vi "GenerateLeftRight.vi"(10 "TrackWidth":dbl=20.0, 11 "SmoothPath":dbl[][](array[numeric])) -> (1 "Right":dbl[][](array[numeric]), 2 "Left":dbl[][](array[numeric]), 3 "Heading":dbl[](array[numeric]))   [LabVIEW 2016]
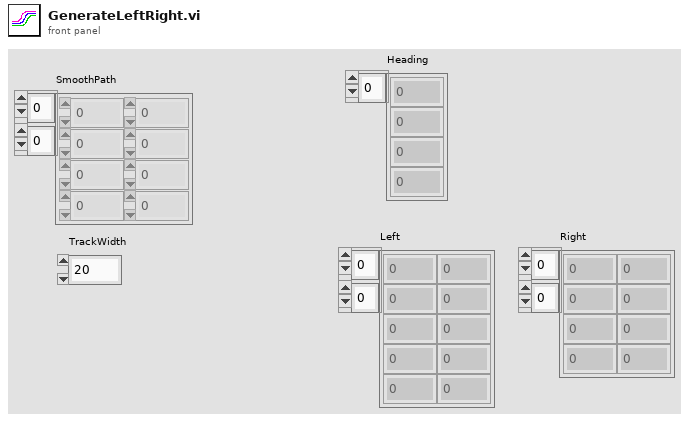
[diagram p1: front panel]
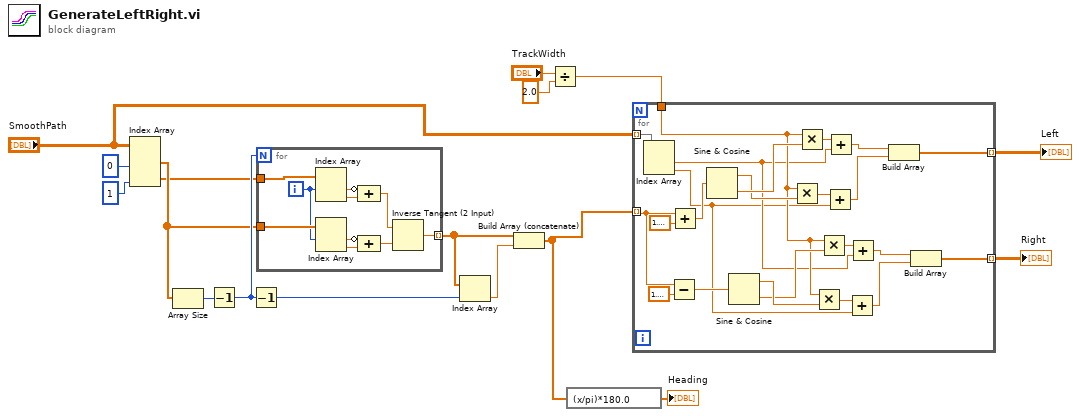
[diagram p0: block diagram]
diagram:
  n1 = Index Array(array="SmoothPath", index (col) #1=0 ("disabled index (col)"), index (col) #2=1 ("index (col)")) -> (element #1=w12:dbl[], element #2=w11:dbl[])  [unwired: 2 in]
  n2 = Array Size(array=w12) -> (size(s)=w16:i32)
  n3 = Decrement(x=w16) -> (x-1=w14:i32)
  n4 = Decrement(x=w14) -> (x-1=w13:i32)
  n5 = for {
    N: w14 -> [_]
    tunnel: w12 -> [w27]
    tunnel: w11 -> [w26]
    tunnel: [w19] -> w3 mode=indexing
    i -> [w18]
    n6 = Index Array(array=w26, index #1=w18) -> (element #1=w24:dbl, element #2=w25:dbl)  [unwired: 1 in]
    n7 = Index Array(array=w27, index #1=w18) -> (element #1=w22:dbl, element #2=w23:dbl)  [unwired: 1 in]
    n8 = Compound Arithmetic op=ADD(invert w24, w25) -> (w21:dbl)
    n9 = Compound Arithmetic op=ADD(invert w22, w23) -> (w20:dbl)
    n10 = Inverse Tangent (2 Input)(1:w20, 2:w21) -> (0:w19:dbl)
  }
  n11 = Index Array(array=w3, index=w13) -> (element=w2:dbl)
  n12 = Build Array (concatenate)(w3, w2) -> (w1:dbl[])
  n13 = Divide(x="TrackWidth", y=2.0) -> (x/y=w8:dbl)
  n14 = expression code="(x/pi)*180.0" ("radians to degrees")(w1) -> (→"Heading":dbl[])
  n15 = for {
    tunnel: w1 -> [w32] mode=indexing
    tunnel: w8 -> [w31]
    tunnel: "SmoothPath" -> [w33] mode=indexing
    tunnel: [w42] -> w6 mode=indexing
    tunnel: [w30] -> w5 mode=indexing
    n16 = Index Array(array=w33) -> (element #1=w29:dbl, element #2=w28:dbl)  [unwired: 2 in]
    n17 = Subtract(x=w32, y=1.5707963267948966) -> (x-y=w35:dbl)
    n18 = Add(x=w32, y=1.5707963267948966) -> (x+y=w49:dbl)
    n19 = Sine & Cosine(0:w49) -> (1:w45:dbl, 2:w46:dbl)
    n20 = Sine & Cosine(0:w35) -> (1:w39:dbl, 2:w38:dbl)
    n21 = Multiply(x=w31, y=w45) -> (x*y=w44:dbl)
    n22 = Multiply(x=w31, y=w46) -> (x*y=w48:dbl)
    n23 = Multiply(x=w31, y=w39) -> (x*y=w40:dbl)
    n24 = Multiply(x=w31, y=w38) -> (x*y=w36:dbl)
    n25 = Add(x=w44, y=w28) -> (x+y=w43:dbl)
    n26 = Add(x=w48, y=w29) -> (x+y=w47:dbl)
    n27 = Add(x=w40, y=w28) -> (x+y=w41:dbl)
    n28 = Add(x=w36, y=w29) -> (x+y=w37:dbl)
    n29 = Build Array(w47, w43) -> (w42:dbl[])
    n30 = Build Array(w37, w41) -> (w30:dbl[])
  }
  "Left" <- w6
  "Right" <- w5
